vi "TestInvalidSubpanelRefnum_ErrorOut.vi"(8 "error in (no error)":errorcluster, 11 "TestCase in":refnum<class "TestProtectedSubpanel.lvclass">) -> (0 "error out":errorcluster, 3 "TestCase out":refnum<class "TestProtectedSubpanel.lvclass">)   [LabVIEW 2015, in "TestProtectedSubpanel.lvclass"]
uses:
  TestProtectedSubpanel.lvclass
  ProtectedSubpanel.lvclass
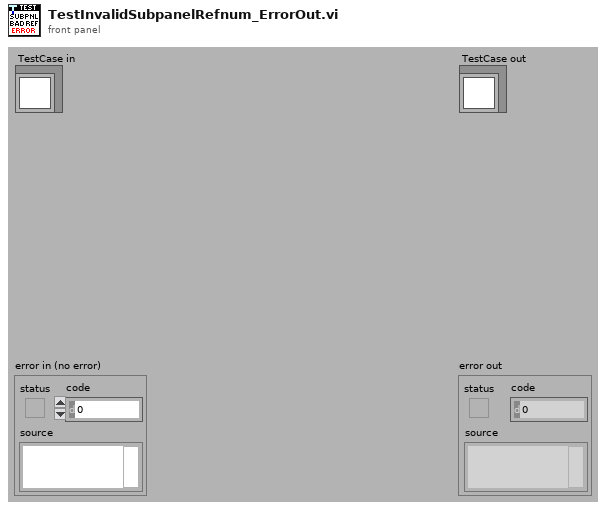
[diagram p1: front panel]
types:
  T1 = typedef "ProtectedSubpanel.lvlib/ProtectedSubpanel.lvclass/Protected Subpanel Reference.ctl" = refnum<data-value>
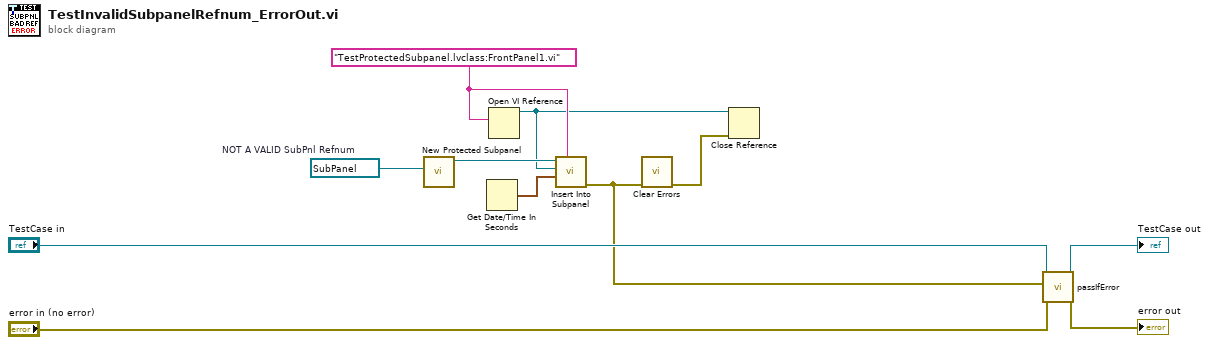
[diagram p0: block diagram]
diagram:
  w4 = refnum<vi> refnum  # NOT A VALID SubPnl Refnum
  w5 = "TestProtectedSubpanel.lvclass:FrontPanel1.vi"
  n1 = call "New Protected Subpanel.vi"("SubPnl Refnum"=w4) -> ("Protected Subpanel"=w7:T1)  [unwired: 9 in, 1 out]
  n2 = Get Date/Time In Seconds() -> (seconds since 1Jan1904=w6:timestamp)
  n3 = Open VI Reference(vi path=w5) -> (vi reference=w3:refnum<vi>)  [unwired: 5 in, 1 out]
  n4 = call "Insert Into Subpanel.vi"("Viewable Name"=w5, "Insertion Request Time"=w6, "VI Refnum"=w3, "Protected Subpanel"=w7) -> ("error out"=w2:errorcluster)  [unwired: 6 in, 1 out]
  n5 = call <vilib>:"Clear Errors.vi"("error in (no error)"=w2) -> ("error out"=w1:errorcluster)  [unwired: 5 in, 1 out]
  n6 = Close Reference(reference=w3, error in (no error)=w1) -> ()  [unwired: 1 out]
  n7 = call-dynamic "passIfError.vi"("error in (no error)"="error in (no error)", "error"=w2, "TestCase in"="TestCase in") -> ("error out"=→"error out":errorcluster, "TestCase out"=→"TestCase out":refnum<class "TestProtectedSubpanel.lvclass">)  [unwired: 7 in]
